vi "Write DAQ FIFO Direct Dispatch.vi"(6 "FIFO Timestamps":T2, 8 "error in (no error)":errorcluster, 9 "Timeout (ms)":i32=100, 10 "DAQ In":T1[](array[typedef]), 11 "CIFTag in":refnum<class "CIFChannels.lvclass">) -> (0 "error out":errorcluster, 1 "timed out?":bool, 2 "DAQ Out":T1[](array[typedef]), 3 "CIFTag out":refnum<class "CIF_NIChn_Fifo_DAQ.lvclass">)   [LabVIEW 2021, in "CIF_NIChn_Fifo_DAQ.lvclass"]
uses:
  CIF_NIChn_Fifo_DAQ.lvclass
  CIFChannels/CIFChannels.lvclass
  ChannelCommon/typedef/TimeStamps.ctl
  ChannelCommon/ChannelCommon.lvlib
  ChannelCommon/typedef/Datatype Waveform.ctl
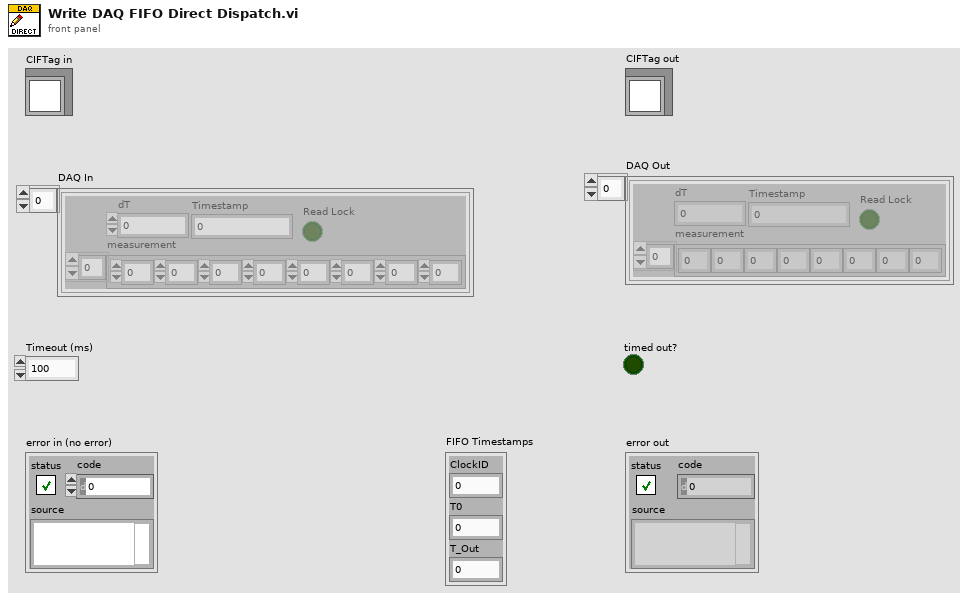
[diagram p1: front panel]
types:
  T1 = typedef "ChannelCommon.lvlib/Datatype Waveform.ctl" = cluster{"measurement":dbl[], "dT":dbl, "Timestamp":i64, "Read Lock":bool}
  T2 = typedef "ChannelCommon.lvlib/TimeStamps.ctl" = cluster{"ClockID":u8, "T0":i64, "T_Out":i64}
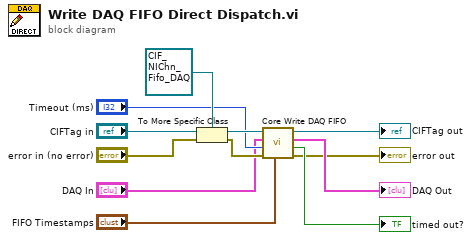
[diagram p0: block diagram]
diagram:
  n1 = To More Specific Class(target class=refnum<class "CIF_NIChn_Fifo_DAQ.lvclass"> refnum ("CIFTag in"), reference="CIFTag in", error in="error in (no error)") -> (specific class reference=w9:refnum<class "CIF_NIChn_Fifo_DAQ.lvclass">, error out=w8:errorcluster)
  n2 = call "Core Write DAQ FIFO.vi"("FIFO Timestamps"="FIFO Timestamps", "error in (no error)"=w8, "Timeout (ms)"="Timeout (ms)", "DAQ In"="DAQ In", "CIFTag in"=w9) -> ("error out"=→"error out":errorcluster, "timed out?"=→"timed out?":bool, "DAQ Out"=→"DAQ Out":T1[], "CIFTag out"=→"CIFTag out":refnum<class "CIF_NIChn_Fifo_DAQ.lvclass">)  [unwired: 3 in]
